vi "Get Real Class Name.vi"(8 "error in (no error)":errorcluster, 11 "Selection in":refnum<class "Selection.lvclass">) -> (0 "error out":errorcluster, 2 "Real Class":string, 3 "Selection out":refnum<class "Selection.lvclass">)   [LabVIEW 2017, in "LV Image Editor Framework.lvlib" / "Selection.lvclass"]
uses:
  <vilib>/LIEF/Forms/Selection/Selection.lvclass
  <vilib>/LIEF/Forms/Selection/Selection.lvclass/Selection.ctl
  <vilib>/LIEF/Forms/Selection/Read Selected Shape.vi
  <vilib>/LIEF/Forms/Shape/Shape.lvclass
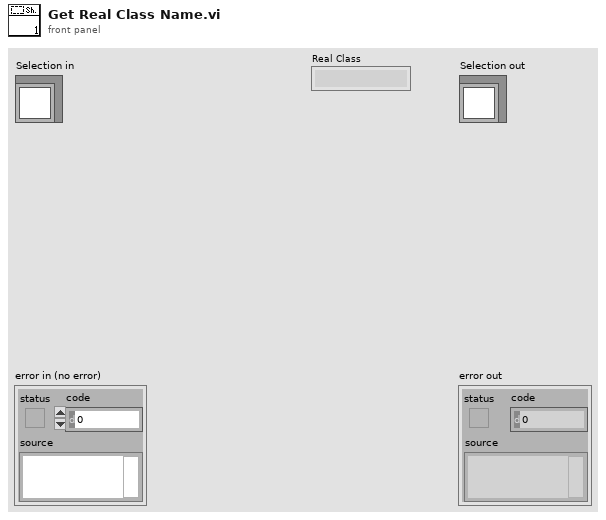
[diagram p1: front panel]
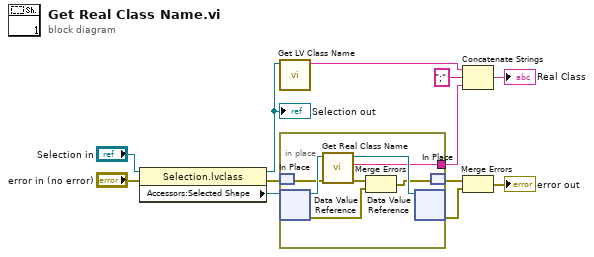
[diagram p0: block diagram]
diagram:
  n1 = property class="Selection.lvclass"(reference="Selection in", error in="error in (no error)") -> (reference out=w5:refnum<class "Selection.lvclass">, error out=w8:errorcluster, "Accessors:Selected Shape"=w11:refnum<data-value>)
  "Selection out" <- w5
  n2 = call <vilib>:"Get LV Class Name.vi"("object"=w5) -> ("class name"=w4:string)  [unwired: 9 in, 1 out]
  n3 = in-place {
    in-place-border: [w13] -> w3
    n4 = in-place-match #1(w8) -> (w15:errorcluster)
    n5 = in-place-dvr #2(w11) -> (w19:refnum<class "Shape.lvclass">, w14:errorcluster)
    n6 = call-dynamic "Get Real Class Name.vi"("error in (no error)"=w15, "Shape in"=w19) -> ("error out"=w16:errorcluster, "Real Class"=w13:string, "Shape out"=w18:refnum<class "Shape.lvclass">)  [unwired: 7 in]
    n7 = Merge Errors(w16, w14) -> (w17:errorcluster)
    n8 = in-place-dvr #2(w18) -> (w6:errorcluster)  [unwired: 1 out]
    n9 = in-place-match #1(w17) -> (w7:errorcluster)
  }
  n10 = Concatenate Strings(w4, ";" ("string"), w3) -> (→"Real Class":string)
  n11 = Merge Errors(w7, w6) -> (→"error out":errorcluster)
